vi "Comments.Add Lockin Description.vi"(7 "error in (no error)":errorcluster, 10 "Control Experiment":refnum<class "Control Experiment.lvclass">) -> (0 "error out":errorcluster, 3 "Control Experiment out":refnum<class "Control Experiment.lvclass">)   [LabVIEW 2016, in "Control Experiment.lvclass"]
uses:
  Control Experiment.lvclass
  Control Experiment.lvclass/Control Experiment.ctl
panel:
  out "Lockin Comments":string
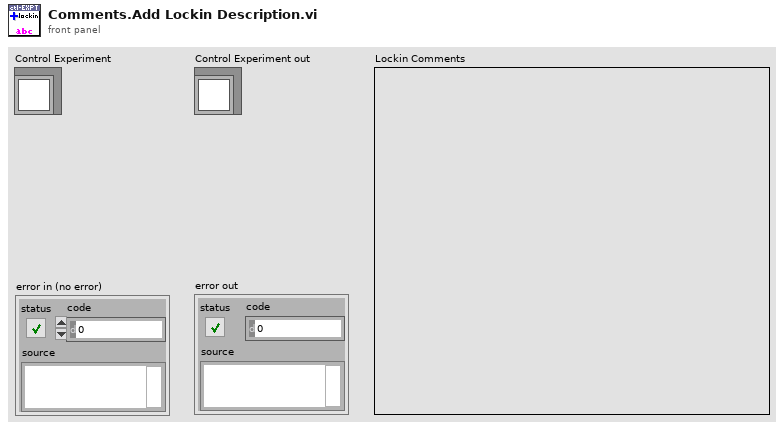
[diagram p1: front panel]
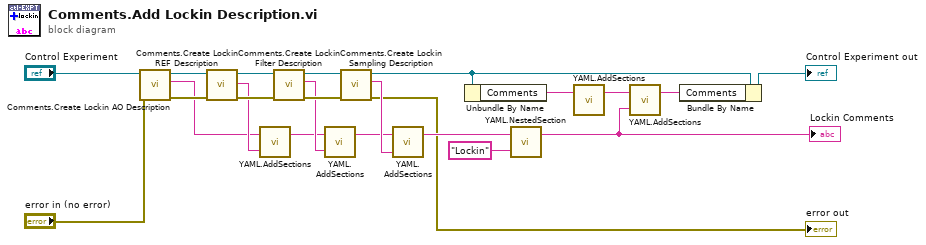
[diagram p0: block diagram]
diagram:
  n1 = call "Comments.Create Lockin AO Description.vi"("error in (no error)"="error in (no error)", "Control Experiment"="Control Experiment") -> ("error out"=w16:errorcluster, "AO Section"=w4:string, "Control Experiment out"=w17:refnum<class "Control Experiment.lvclass">)  [unwired: 6 in]
  n2 = call "Comments.Create Lockin REF Description.vi"("error in (no error)"=w16, "Control Experiment"=w17) -> ("error out"=w14:errorcluster, "REF Section"=w6:string, "Control Experiment out"=w15:refnum<class "Control Experiment.lvclass">)  [unwired: 6 in]
  n3 = call "YAML.AddSections.vi"("Section 2"=w6, "Section 1"=w4) -> ("Output"=w5:string)  [unwired: 1 in]
  n4 = call "Comments.Create Lockin Filter Description.vi"("error in (no error)"=w14, "Control Experiment"=w15) -> ("error out"=w12:errorcluster, "Filter Section"=w7:string, "Control Experiment out"=w13:refnum<class "Control Experiment.lvclass">)  [unwired: 6 in]
  n5 = call "YAML.AddSections.vi"("Section 2"=w7, "Section 1"=w5) -> ("Output"=w8:string)  [unwired: 1 in]
  n6 = call "Comments.Create Lockin Sampling Description.vi"("error in (no error)"=w12, "Control Experiment"=w13) -> ("error out"=→"error out":errorcluster, "Sampling Section"=w9:string, "Control Experiment out"=w18:refnum<class "Control Experiment.lvclass">)  [unwired: 6 in]
  n7 = call "YAML.AddSections.vi"("Section 2"=w9, "Section 1"=w8) -> ("Output"=w3:string)  [unwired: 1 in]
  n8 = Unbundle By Name(w18) -> ("Comments"=w22:string)
  n9 = call "YAML.NestedSection.vi"("Section Key"="Lockin" ("string"), "Nested Section"=w3) -> ("String"=w10:string)  [unwired: 1 in]
  "Lockin Comments" <- w10
  n10 = call "YAML.AddSections.vi"("Section 1"=w22) -> ("Output"=w21:string)  [unwired: 2 in]
  n11 = call "YAML.AddSections.vi"("Section 2"=w10, "Section 1"=w21) -> ("Output"=w20:string)  [unwired: 1 in]
  n12 = Bundle By Name(cluster=w18, "Comments"=w20) -> (→"Control Experiment out":refnum<class "Control Experiment.lvclass">)
